vi "Read Shunt Resistor Location.vi"(8 "error in (no error)":errorcluster, 11 "BNT_DAQmx-MCSV-I in":refnum<class "BNT_DAQmx-MCSV-I.lvclass">) -> (0 "error out":errorcluster, 2 "Shunt Resistor Location":i32(ring)=-1 items=["default"=-1, "Internal"=10200, "External"=10167], 3 "BNT_DAQmx-MCSV-I out":refnum<class "BNT_DAQmx-MCSV-I.lvclass">)   [LabVIEW 2021, in "BNT_DAQmx.lvlib" / "BNT_DAQmx-MCSV-I.lvclass"]
doc: "Read shunt resistor location."
uses:
  BNT_DAQmx-MCSV-I.lvclass
  BNT_DAQmx-MCSV-I.lvclass/BNT_DAQmx-MCSV-I.ctl
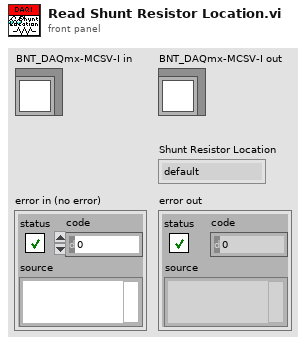
[diagram p1: front panel]
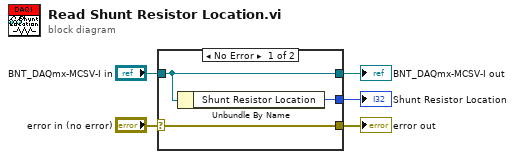
[diagram p0: block diagram]
diagram:
  n1 = case shown="No Error" "error in (no error)" {
    selector: "error in (no error)" -> [w8 w9]
    tunnel: [w8 w9] -> w4
    tunnel: [w7 w10] -> w2
    tunnel: "BNT_DAQmx-MCSV-I in" -> [w7 w10]
    tunnel: [w6 _] -> w1
    frame No Error {
      n2 = Unbundle By Name(w7) -> ("Shunt Resistor Location"=w6:i32)
    }
    frame Error {
    }
  }
  "error out" <- w4
  "BNT_DAQmx-MCSV-I out" <- w2
  "Shunt Resistor Location" <- w1
